vi "Odometry Loop.vi"(6 "error in (no error)":errorcluster) -> ()   [LabVIEW 2018]
uses:
  Typedef/Velocity Data.ctl
  Typedef/Odometry.ctl
  <vilib>/Platform/TimedLoop/XDataNode/wakeup.ctl
  <vilib>/Platform/TimedLoop/XDataNode/XDNodeRunTimeDep.lvlib
  <vilib>/Platform/TimedLoop/XDataNode/nitl_modes.ctl
  <vilib>/Platform/TimedLoop/XDataNode/timing_clust.ctl
  <vilib>/platform/TimedLoop/XDataNode/XDataNode.xnode
  Drive/Pure Pursuit/Pure Pursuit.lvlib
  Drive/Pure Pursuit/Visualization/Current Path.vi
  <vilib>/Rock Robotics/Network Tables/NT Write Numeric Array.vi
  Drive/Pure Pursuit/Typedef/Pure Pursuit Telemetry.ctl
  Drive/Pure Pursuit/Typedef/Path Point.ctl
  <vilib>/Rock Robotics/Network Tables/NT Write Number.vi
panel:
  out "Late Iterations":i16
  out "XY Graph":cluster{dbl[], dbl[]}[](graph)=[{array[1000 elements], array[1000 elements]}, {[-2.247939211922799, 9.450601976465425, 8.114176327244312, -3.5843648611439116, -2.247939211922799], [3.8835413402382706, 1.2106900417960451, -4.638580552398066, -1.9657292539558406, 3.8835413402382706]}, {[0.0, 40.0, 60.0, 100.0], [0.0, 20.0, 80.0, 40.0]}, {array[304 elements], array[304 elements]}, {[7.524752475247524, 1.9801980198019802], [-4.118238955689372, -1.1545613507952672]}, {[-5.727080057823512, -5.705598316147173, -5.641285533198998, -5.534538218672029, -5.386014505257412, -5.196630091037495, -4.967552593902651, -4.700194352798713, -4.396203720187724, -4.057454899406876, -3.686036389581695, -3.28423810933444, -2.8545372786743237, -2.3995831461123918, -1.922180655163488, -1.4252731509367513, -0.9119242334342519, -0.38529886943823066, 0.15135612056157366, 0.6947320800959187, 1.241478915683433, 1.7882257512709472, 2.331601710805292, 2.8682567008050963, 3.3948820648011178, 3.9082309823036177, 4.405138486530354, 4.882540977479257, 5.337495110041189, 5.767195940701306, 6.16899422094856, 6.540412730773742, 6.87916155155459, 7.1831521841655785, 7.450510425269517, 7.679587922404362, 7.86897233662428, 8.017496050038897, 8.124243364565864, 8.18855614751404, 8.210037889190378, 8.18855614751404, 8.124243364565865, 8.017496050038897, 7.86897233662428, 7.679587922404362, 7.450510425269517, 7.18315218416558, 6.879161551554592, 6.540412730773744, 6.168994220948562, 5.76719594070131, 5.337495110041191, 4.882540977479256, 4.405138486530356, 3.9082309823036216, 3.3948820648011195, 2.868256700805095, 2.3316017108052938, 1.788225751270952, 1.2414789156834347, 0.6947320800959172, 0.15135612056157544, -0.3852988694382258, -0.9119242334342501, -1.4252731509367527, -1.9221806551634866, -2.3995831461123878, -2.854537278674323, -3.2842381093344417, -3.686036389581693, -4.057454899406872, -4.396203720187724, -4.700194352798713, -4.967552593902649, -5.196630091037493, -5.386014505257412, -5.534538218672031, -5.641285533198998, -5.705598316147173, -5.727080057823512], [-7.13175642584397, -7.6785032614314845, -8.22187922096583, -8.758534210965633, -9.285159574961655, -9.798508492464155, -10.295415996690892, -10.772818487639794, -11.227772620201726, -11.657473450861843, -12.059271731109098, -12.430690240934279, -12.769439061715127, -13.073429694326116, -13.340787935430054, -13.5698654325649, -13.759249846784815, -13.907773560199434, -14.0145208747264, -14.078833657674576, -14.100315399350915, -14.078833657674576, -14.0145208747264, -13.907773560199434, -13.759249846784817, -13.5698654325649, -13.340787935430054, -13.073429694326116, -12.769439061715127, -12.430690240934279, -12.0592717311091, -11.657473450861843, -11.227772620201728, -10.772818487639796, -10.295415996690892, -9.798508492464155, -9.285159574961655, -8.758534210965635, -8.22187922096583, -7.678503261431485, -7.131756425843971, -6.5850095902564565, -6.041633630722112, -5.504978640722308, -4.978353276726287, -4.465004359223786, -3.9680968549970497, -3.4906943640481467, -3.035740231486214, -2.6060394008260976, -2.2042411205788426, -1.8328226107536638, -1.4940737899728127, -1.1900831573618227, -0.922724916257887, -0.6936474191230433, -0.504263004903124, -0.355739291488506, -0.2489919769615394, -0.18467919401336363, -0.16319745233702498, -0.18467919401336363, -0.24899197696153852, -0.355739291488506, -0.5042630049031231, -0.6936474191230424, -0.9227249162578861, -1.1900831573618218, -1.4940737899728118, -1.832822610753662, -2.2042411205788417, -2.6060394008260923, -3.035740231486211, -3.4906943640481467, -3.9680968549970475, -4.465004359223782, -4.978353276726283, -5.5049786407223085, -6.041633630722109, -6.585009590256451, -7.131756425843968]}]
  out "Drivetrain Chart":T1(graph)
  out "Gyro":dbl(graph)
  out "Encoders":T2(graph)
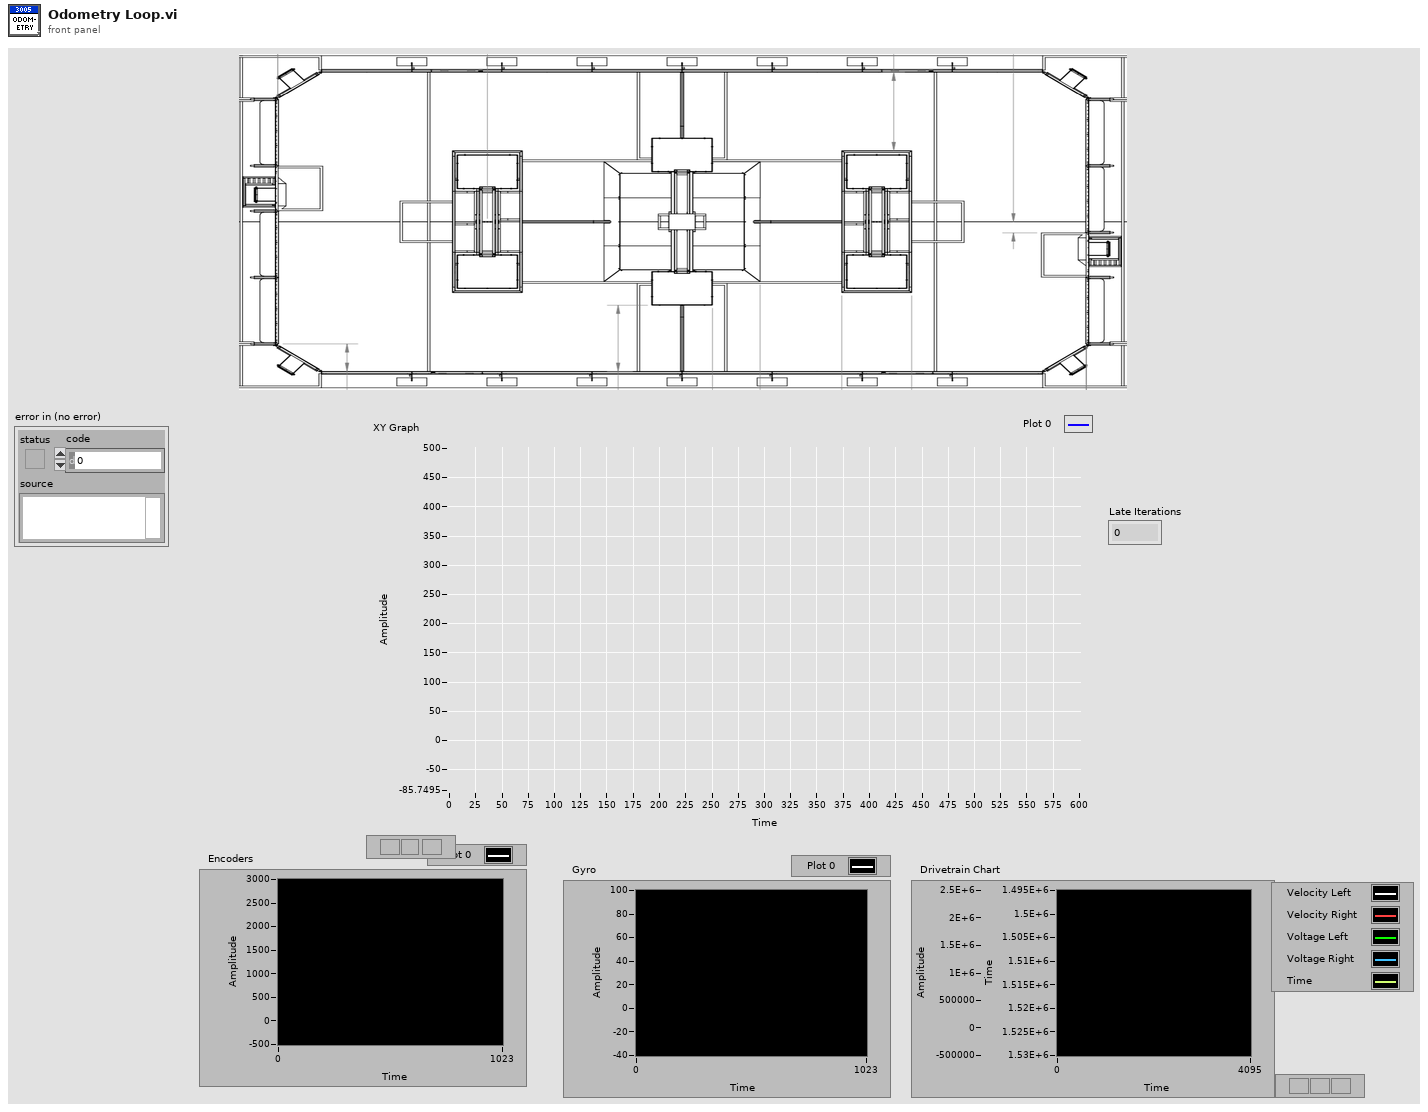
[diagram p1: front panel]
types:
  T1 = cluster{"Left Velocity Raw":sgl, "Right Velocity Raw":sgl, "Voltage":dbl, "Voltage":dbl, "Tick Count(mSec)":u32}
  T2 = cluster{"Left Velocity Raw":sgl, "Right Velocity Raw":sgl}
  T3 = typedef "SPARKMAX6Motor.ctl" = cluster{"FrontLeftMaster":T4, "FrontLeftSlave1":T4, "FrontLeftSlave2":T4, "FrontRightMaster":T4, "FrontRightSlave1":T4, "FrontRightSlave2":T4}
  T4 = typedef "WPI_MotorControlDeviceRef.ctl" = cluster{"DeviceStatus":errorcluster, "Type":T5, "PWM":cluster{"PWM Channel":T6, "DeadBand":T7}, "CAN":cluster{"Device Number":u8, "SetOutput VI Ref":variant, "GetOutput VI Ref":variant, "Enable VI Ref":variant, "Disable VI Ref":variant, "Data":variant}, "Invert":bool, "DIO PWM":cluster{"PWM \"Enable\" Channel":T6, "DIOChannel":T8, "PWM Rate":dbl}}
  T5 = typedef "WPI_MotorControlType.ctl" = enum16{"PWM", "CAN", "DIO PWM"}
  T6 = typedef "FPGA_DIOPWMChannel.ctl" = enum8{"PWM 0", "PWM 1", "PWM 2", "PWM 3", "PWM 4", "PWM 5", "PWM 6", "PWM 7", "PWM 8", "PWM 9", "PWM MXP 0", "PWM MXP 1", "PWM MXP 2", "PWM MXP 3", "PWM MXP 4", "PWM MXP 5", "PWM MXP 6", "PWM MXP 7", "PWM MXP 8", "PWM MXP 9", "Invalid"}
  T7 = typedef "WPI_PWMDeadband.ctl" = cluster{"Name":string, "maxPositivePwm":i32, "minPositivePwm":i32, "centerPwm":i32, "maxNegativePwm":i32, "minNegativePwm":i32, "angularRange":u16}
  T8 = typedef "FPGA_DIOChannel.ctl" = enum8{"DIO 0", "DIO 1", "DIO 2", "DIO 3", "DIO 4", "DIO 5", "DIO 6", "DIO 7", "DIO 8", "DIO 9", "DIO MXP 0", "DIO MXP 1", "DIO MXP 2", "DIO MXP 3", "DIO MXP 4", "DIO MXP 5", "DIO MXP 6", "DIO MXP 7", "DIO MXP 8", "DIO MXP 9", "DIO MXP 10", "DIO MXP 11", "DIO MXP 12", "DIO MXP 13", "DIO MXP 14", "DIO MXP 15", "SPI Port CS1", "SPI Port CS2", "SPI Port CS3", "SPI Port MISO", "SPI Port MOSI", "Invalid"}
  T9 = typedef "Pure Pursuit.lvlib/Pure Pursuit Telemetry.ctl" = cluster{"Target Point":T10, "Close Point":T10, "Curvature":dbl, "index out":i32}
  T10 = typedef "Pure Pursuit.lvlib/Path Point.ctl" = cluster{"x":dbl, "y":dbl, "heading":dbl, "curvature":dbl, "total distance":dbl, "velocity expected":dbl}
  T11 = typedef "Odometry.ctl" = cluster{"x":dbl, "y":dbl, "theta":dbl, "Left Encoder":dbl, "Right Encoder":dbl, "Late Iterations":i16}
  T12 = typedef "Velocity Data.ctl" = cluster{"Right Velocity Raw":sgl, "Left Velocity Raw":sgl}
  T13 = typedef "WPI_GyroDevRef.ctl" = cluster{"DevStatus":errorcluster, "Analog Channel":T14, "Gain (VoltsPerDegree/Second)":dbl, "Gyro Type":enum16{"Analog", "XRS450"}, "Handle":i32, "SPI Bus":T15, "Device Found":bool, "Sample Rate":dbl, "Calibrate On Open":bool, "Offset":dbl}
  T14 = typedef "FPGA_AIChannel.ctl" = enum8{"AI 0", "AI 1", "AI 2", "AI 3", "AI MXP 0", "AI MXP 1", "AI MXP 2", "AI MXP 3", "Invalid"}
  T15 = typedef "spi_bus.ctl" = enum16{"SPI On-Board, CS0", "SPI On-Board, CS1", "SPI On-Board, CS2", "SPI On-Board, CS3", "SPI MXP", "Invalid"}
  T16 = typedef "XDNodeRunTimeDep.lvlib/timing_clust.ctl" = cluster{"Expected End [f-1]":u64, "Actual End [f-1]":u64, "Finished Late? [f-1]":bool, "Expected End [i-1]":u64, "Actual End [i-1]":u64, "Finished Late? [i-1]":bool, "Expected Start [i]":u64, "Actual Start [i]":u64, "Expected Start [f]":u64, "Actual Start [f]":u64, "Source Name":string, "Structure Name":string, "Period":i64, "Deadline":i64, "Offset":i64, "Start":i64, "Priority":i32, "Timeout":i32, "Mode":T17, "Wakeup Reason":T18, "Error":errorcluster, "Source Type":string, "Secondary Source Type":string, "Global End Time":u64, "Global Start Time":u64, "Frame Duration":u64, "Iteration Duration":u64, "Assigned CPU":i32, "I/O Scan Engine Mode":u32}
  T17 = typedef "XDNodeRunTimeDep.lvlib/nitl_modes.ctl" = enum32{"No Change", "Process missed periods, maintain original phase", "Discard missed periods, maintain original phase", "Process missed periods, ignore original phase", "Discard missed periods, ignore original phase"}
  T18 = typedef "XDNodeRunTimeDep.lvlib/wakeup.ctl" = enum32{"Normal", "Aborted", "Asynchronous wakeup", "Timing source error", "Timed loop error", "Timeout"}
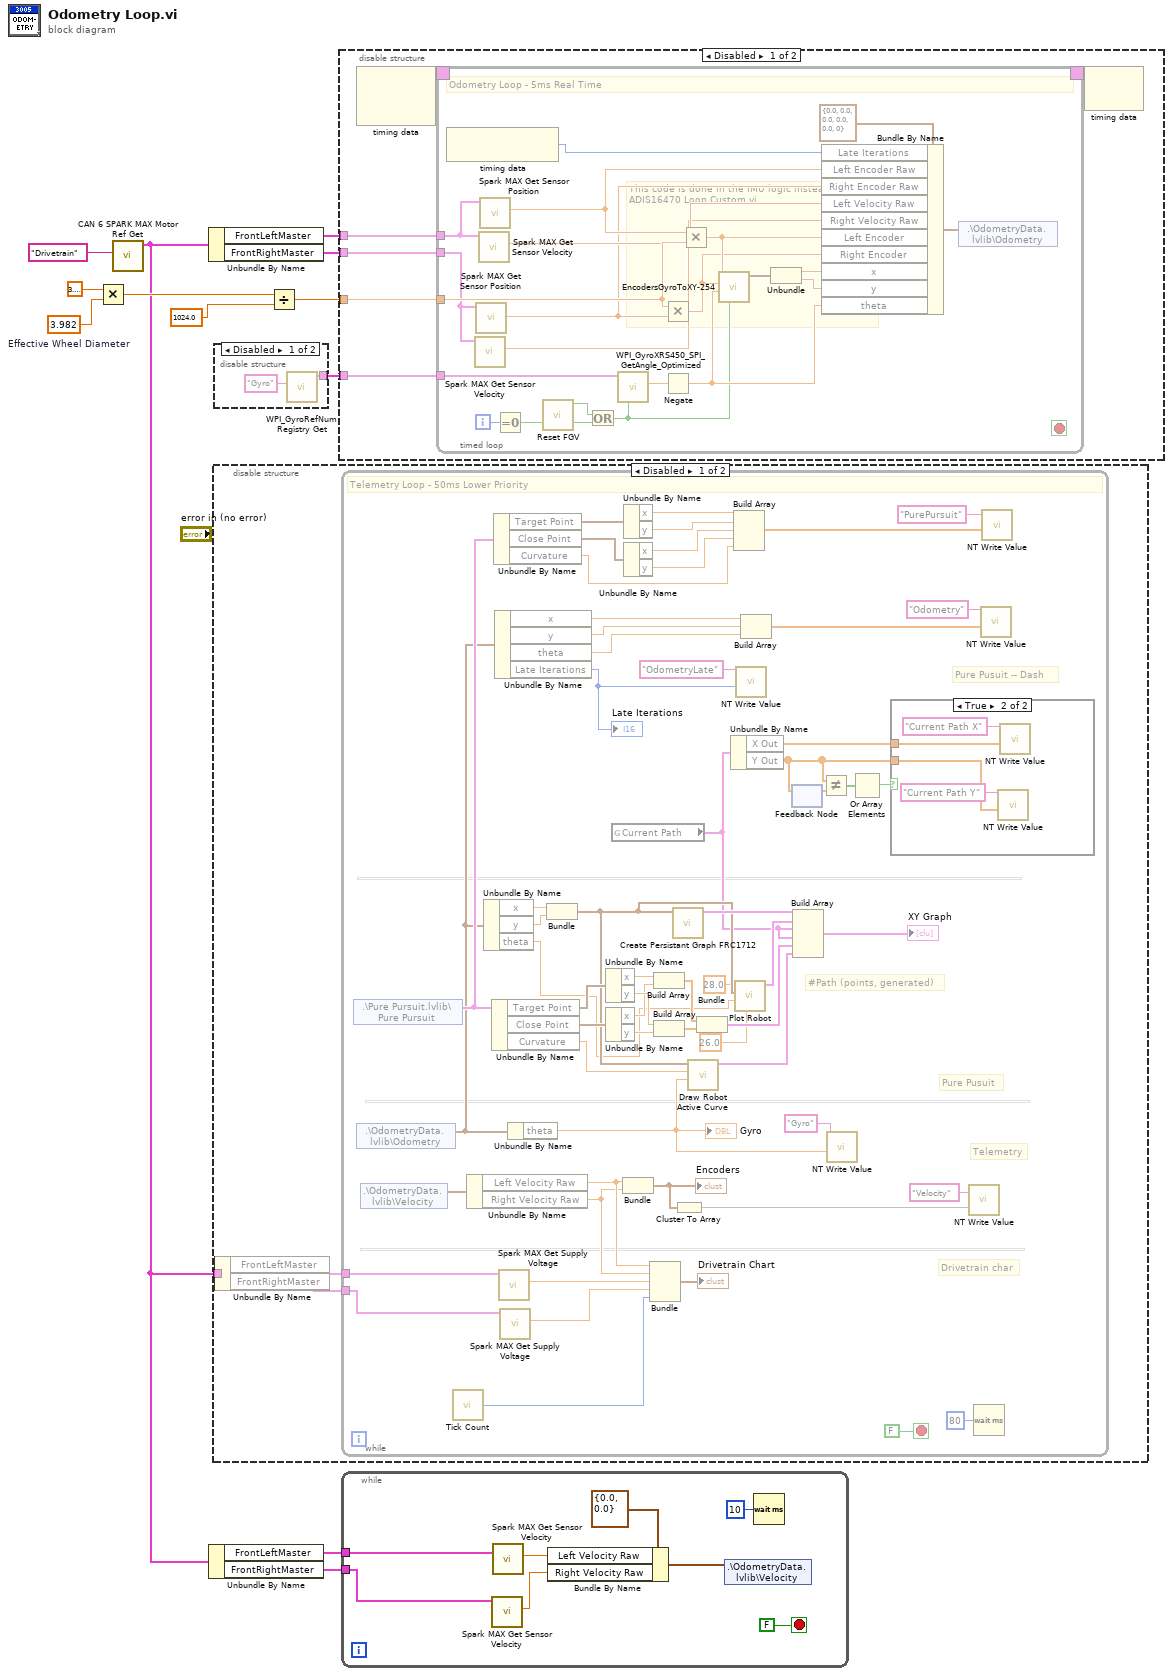
[diagram p0: block diagram]
diagram:
  w8 = 3.982  # Effective Wheel Diameter
  # "This code is done in the IMU logic instead: ADIS16470 Loop Custom.vi"
  n1 = Multiply(x=3.141592653589793, y=w8) -> (x*y=w6:dbl)
  n2 = call "CAN 6 SPARK MAX Motor Ref Get.vi"("refnum name"="Drivetrain") -> ("TalonSRX6MotorRef out"=w3:T3)  [unwired: 9 in, 1 out]
  n3 = Unbundle By Name(w3) -> ("FrontLeftMaster"=w11:T4, "FrontRightMaster"=w12:T4)
  n4 = Unbundle By Name(w3) -> ("FrontLeftMaster"=w2:T4, "FrontRightMaster"=w1:T4)
  n5 = disable-structure shown="Disabled" {
    disable-tunnel: w3 -> [w13 _]
    frame Disabled {
      n6 = Unbundle By Name(w13) -> ("FrontLeftMaster"=w15:T4, "FrontRightMaster"=w14:T4)
      n7 = while {
        tunnel: w15 -> [w22]
        tunnel: w14 -> [w19]
        stop <- FALSE stop-if-true
        # "Pure Pusuit -- Dash"
        # "Telemetry"
        # "Drivetrain char"
        # "Pure Pusuit"
        # "#Path (points, generated)"
        # "Telemetry Loop - 50ms Lower Priority"
        n8 = shared-variable ".\\Pure Pursuit.lvlib\\Pure Pursuit"() -> (w44:T9)  [unwired: 1 in, 1 out]
        n9 = shared-variable ".\\OdometryData.lvlib\\Odometry"() -> (w35:T11)  [unwired: 1 in, 1 out]
        n10 = shared-variable ".\\OdometryData.lvlib\\Velocity"() -> (w18:T12)  [unwired: 1 in, 1 out]
        n11 = call "Tick Count"() -> ("Tick Count(mSec)"=w50:u32)
        n12 = Unbundle By Name(w18) -> ("Left Velocity Raw"=w17:sgl, "Right Velocity Raw"=w16:sgl)
        n13 = Unbundle By Name(w35) -> ("x"=w70:dbl, "y"=w69:dbl, "theta"=w52:dbl)
        n14 = Unbundle By Name(w44) -> ("Target Point"=w59:T10, "Close Point"=w58:T10, "Curvature"=w57:dbl)
        n15 = Unbundle By Name(w44) -> ("Target Point"=w43:T10, "Close Point"=w42:T10, "Curvature"=w37:dbl)
        n16 = Unbundle By Name(w35) -> ("x"=w34:dbl, "y"=w33:dbl, "theta"=w32:dbl, "Late Iterations"=w23:i16)
        "Late Iterations" <- w23
        n17 = call <vilib>:"Spark MAX Get Supply Voltage.vi"("MotorControlDevRef in"=w22) -> ("Voltage"=w21:dbl)  [unwired: 7 in, 3 out]
        n18 = call <vilib>:"Spark MAX Get Supply Voltage.vi"("MotorControlDevRef in"=w19) -> ("Voltage"=w20:dbl)  [unwired: 7 in, 3 out]
        n19 = Unbundle By Name(w35) -> ("theta"=w55:dbl)
        "Gyro" <- w55
        n20 = Bundle("x"=w70, "y"=w69) -> (w54:cluster{"x":dbl, "y":dbl})  [unwired: 1 in]
        n21 = Unbundle By Name(w59) -> ("x"=w66:dbl, "y"=w65:dbl)
        n22 = Unbundle By Name(w58) -> ("x"=w62:dbl, "y"=w61:dbl)
        n23 = global read "Current Path.vi" "Current Path"() -> (w30:cluster{"X Out":dbl[], "Y Out":dbl[]})
        n24 = Bundle("Left Velocity Raw"=w17, "Right Velocity Raw"=w16) -> (w48:T2)  [unwired: 1 in]
        "Encoders" <- w48
        n25 = Unbundle By Name(w43) -> ("x"=w41:dbl, "y"=w40:dbl)
        n26 = Unbundle By Name(w42) -> ("x"=w39:dbl, "y"=w38:dbl)
        n27 = Bundle("Left Velocity Raw"=w17, "Right Velocity Raw"=w16, "Voltage"=w21, "Voltage"=w20, "Tick Count(mSec)"=w50) -> (→"Drivetrain Chart":T1)  [unwired: 1 in]
        n28 = Build Array(w66, w62) -> (w63:dbl[])
        n29 = Build Array(w65, w61) -> (w64:dbl[])
        n30 = call "Create Persistant Graph FRC1712.vi"("XY"=w54) -> ("Graph Plot"=w73:cluster{dbl[], dbl[]})  [unwired: 10 in]
        n31 = Cluster To Array(cluster=w48) -> (array=w47:sgl[])
        n32 = call "Draw Robot Active Curve.vi"("theta"=w55, "Curvature"=w57, "Cluster"=w54) -> ("circle"=w56:cluster{dbl[], dbl[]})  [unwired: 8 in]
        n33 = Bundle(w63, w64) -> (w60:cluster{dbl[], dbl[]})  [unwired: 1 in]
        n34 = Unbundle By Name(w30) -> ("X Out"=w29:dbl[], "Y Out"=w27:dbl[])
        n35 = Build Array(w41, w40, w39, w38, w37) -> (w36:dbl[])
        n36 = call "Plot Robot.vi"("Length"=26.0, "Angle"=w52, "Location"=w54, "Width"=28.0) -> ("Cluster"=w67:cluster{"X Out":dbl[], "Y Out":dbl[]})  [unwired: 7 in]
        n37 = call-poly <vilib>:"NT Write Value.vi"("Numeric"=w23, "Name"="OdometryLate") -> ()  [unwired: 9 in, 1 out]
        n38 = Build Array(w34, w33, w32) -> (w31:dbl[])
        n39 = feedback-in #1(w27) -> ()
        n40 = feedback #1() -> (w28:dbl[])  [unwired: 1 in]
        n41 = Build Array(w73, w67, w30, w30, w60, w56) -> (→"XY Graph":cluster{"X Out":dbl[], "Y Out":dbl[]}[])
        n42 = Not Equal?(x=w27, y=w28) -> (x != y?=w26:bool[])
        n43 = call-poly <vilib>:"NT Write Value.vi"("Numeric"=w55, "Name"="Gyro") -> ()  [unwired: 9 in, 1 out]
        n44 = Or Array Elements(Boolean array=w26) -> (logical OR=w25:bool)
        n45 = case shown="True" w25 {
          tunnel: w27 -> [_ w77]
          tunnel: w29 -> [_ w76]
          frame False {
          }
          frame True {
            n46 = call-poly <vilib>:"NT Write Value.vi"("Numeric Array"=w77, "Name"="Current Path Y") -> ()  [unwired: 9 in, 1 out]
            n47 = call-poly <vilib>:"NT Write Value.vi"("Numeric Array"=w76, "Name"="Current Path X") -> ()  [unwired: 9 in, 1 out]
          }
        }
        n48 = call-poly <vilib>:"NT Write Value.vi"("Numeric Array"=w47, "Name"="Velocity") -> ()  [unwired: 9 in, 1 out]
        n49 = Wait (ms)(milliseconds to wait=u32 80) -> ()  [unwired: 1 out]
        n50 = call-poly <vilib>:"NT Write Value.vi"("Numeric Array"=w31, "Name"="Odometry") -> ()  [unwired: 9 in, 1 out]
        n51 = call-poly <vilib>:"NT Write Value.vi"("Numeric Array"=w36, "Name"="PurePursuit") -> ()  [unwired: 9 in, 1 out]
      }
    }
    frame Enabled {
    }
  }
  n52 = disable-structure shown="Disabled" {
    disable-tunnel: [w81 _] -> w9
    frame Disabled {
      n53 = call <vilib>:"WPI_GyroRefNum Registry Get.vi"("refnum name"="Gyro") -> ("GyroDevRef"=w81:T13)  [unwired: 9 in, 1 out]
    }
    frame Enabled {
    }
  }
  n54 = Divide(x=w6, y=1024.0) -> (x/y=w4:dbl)
  n55 = disable-structure shown="Disabled" {
    disable-tunnel: w12 -> [w85 _]
    disable-tunnel: w11 -> [w84 _]
    disable-tunnel: w9 -> [w83 _]
    disable-tunnel: w4 -> [w82 _]
    frame Disabled {
      n56 = node-c288() -> (w87:T16)  [unwired: 2 in]
      n57 = timed-loop {
        timing: w87 -> [_]
        timing-out: [_] -> w86
        tunnel: w83 -> [w100]
        tunnel: w84 -> [w93]
        tunnel: w85 -> [w90]
        tunnel: w82 -> [w98]
        i -> [w109]
        stop <- _ stop-if-true
        # "Odometry Loop - 5ms Real Time"
        n58 = node-c288() -> (w94:i64)  [unwired: 1 in]
        n59 = call <vilib>:"Spark MAX Get Sensor Velocity.vi"("MotorControlDevRef in"=w90) -> ("Sensor Velocity"=w88:dbl)  [unwired: 7 in, 3 out]
        n60 = call <vilib>:"Spark MAX Get Sensor Position.vi"("MotorControlDevRef in"=w90) -> ("Sensor Position"=w89:dbl)  [unwired: 7 in, 3 out]
        n61 = call <vilib>:"Spark MAX Get Sensor Velocity.vi"("MotorControlDevRef in"=w93) -> ("Sensor Velocity"=w91:dbl)  [unwired: 7 in, 3 out]
        n62 = call <vilib>:"Spark MAX Get Sensor Position.vi"("MotorControlDevRef in"=w93) -> ("Sensor Position"=w92:dbl)  [unwired: 7 in, 3 out]
        n63 = Equal To 0?(x=w109) -> (x = 0?=w96:bool)
        n64 = call "Reset FGV.vi"() -> ("Reset?"=w97:bool)  [unwired: 11 in]
        n65 = Or(x=w97, y=w96) -> (x .or. y?=w95:bool)
        n66 = call "WPI_GyroXRS450_SPI_GetAngle_Optimized.vi"("Reset?"=w95, "GyroDevRef"=w100) -> ("Angle"=w99:dbl)  [unwired: 6 in, 3 out]
        n67 = Multiply(x=w98, y=w89) -> (x*y=w101:dbl)
        n68 = Negate(x=w99) -> (-x=w104:dbl)
        n69 = Multiply(x=w92, y=w98) -> (x*y=w102:dbl)
        n70 = call "EncodersGyroToXY-254.vi"("Reset"=w95, "Angle (degrees)"=w104, "Right Distance"=w101, "Left Distance"=w102) -> ("Location"=w107:cluster{"X":dbl, "Y":dbl})  [unwired: 7 in]
        n71 = Unbundle(w107) -> ("X"=w106:dbl, "Y"=w105:dbl)
        n72 = Bundle By Name(cluster=T11 {"x"=0.0, "y"=0.0, "theta"=0.0, "Left Encoder"=0.0, "Right Encoder"=0.0, "Late Iterations"=0} ("Odometry"), "Late Iterations"=w94, "Left Encoder Raw"=w92, "Right Encoder Raw"=w89, "Left Velocity Raw"=w91, "Right Velocity Raw"=w88, "Left Encoder"=w102, "Right Encoder"=w101, "x"=w106, "y"=w105, "theta"=w104) -> (w103:T11)
        n73 = shared-variable ".\\OdometryData.lvlib\\Odometry"(w103) -> ()  [unwired: 1 in, 1 out]
      }
      n74 = node-c288(w86) -> ()  [unwired: 1 out]
    }
    frame Enabled {
    }
  }
  n75 = while {
    tunnel: w2 -> [w120]
    tunnel: w1 -> [w119]
    stop <- FALSE stop-if-true
    n76 = call <vilib>:"Spark MAX Get Sensor Velocity.vi"("MotorControlDevRef in"=w119) -> ("Sensor Velocity"=w118:dbl)  [unwired: 7 in, 3 out]
    n77 = call <vilib>:"Spark MAX Get Sensor Velocity.vi"("MotorControlDevRef in"=w120) -> ("Sensor Velocity"=w117:dbl)  [unwired: 7 in, 3 out]
    n78 = Bundle By Name(cluster=T12 {"Right Velocity Raw"=0.0, "Left Velocity Raw"=0.0} ("Velocity"), "Left Velocity Raw"=w117, "Right Velocity Raw"=w118) -> (w116:T12)
    n79 = shared-variable ".\\OdometryData.lvlib\\Velocity"(w116) -> ()  [unwired: 1 in, 1 out]
    n80 = Wait (ms)(milliseconds to wait=u32 10) -> ()  [unwired: 1 out]
  }
